vi "http transmit response.vi"(8 "error in":errorcluster, 10 "application request":T1, 11 "tcp connection":refnum<k5>) -> (0 "error out":errorcluster)   [LabVIEW 2013]
uses:
  http response.ctl
  http response packet type.ctl
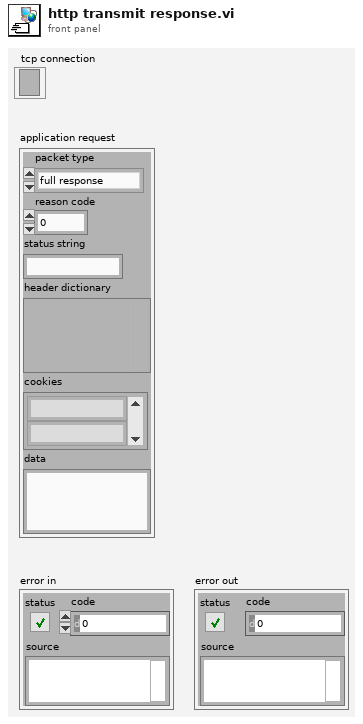
[diagram p1: front panel]
types:
  T1 = typedef "http response.ctl" = cluster{"packet type":T2, "reason code":u16, "status string":string, "header dictionary":variant, "cookies":string[], "data":string}
  T2 = typedef "http response packet type.ctl" = enum16{"full response", "header only", "data only", "last data"}
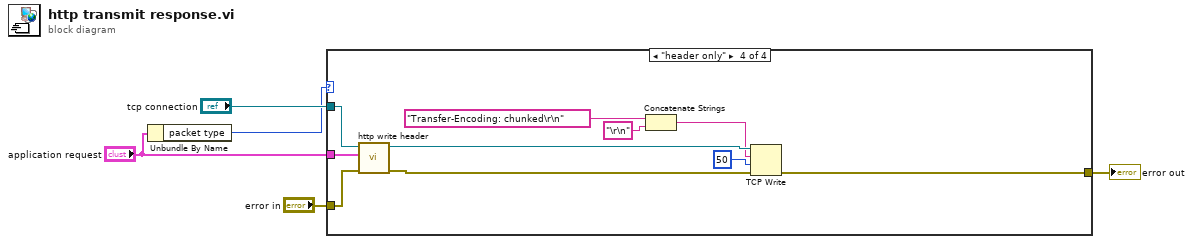
[diagram p0: block diagram]
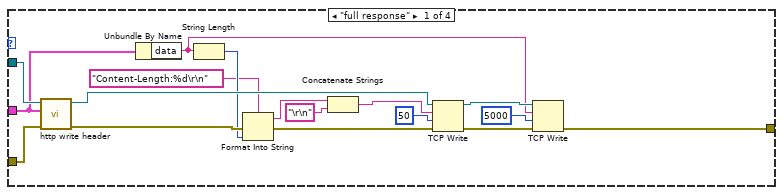
[diagram p2: hidden frame]
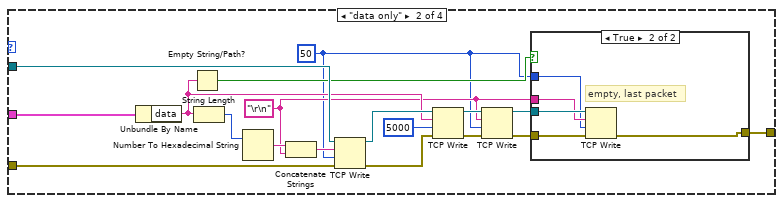
[diagram p3: hidden frame]
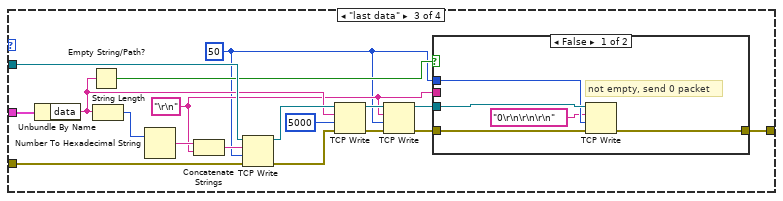
[diagram p5: hidden frame]
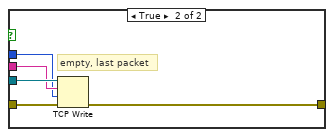
[diagram p6: hidden frame]
diagram:
  n1 = Unbundle By Name("application request") -> ("packet type"=w1:T2)
  n2 = case shown="\"header only\"" w1 {
    tunnel: "tcp connection" -> [w22 w35 w59 w84]
    tunnel: [w12 w25 w49 w79] -> w4
    tunnel: "error in" -> [w9 w40 w64 w81]
    tunnel: "application request" -> [w8 w37 w61 w80]
    frame "full response" {
      n3 = call "http write header.vi"("error in (no error)"=w9, "application request"=w8, "TCP Network Connection in"=w22) -> ("error out"=w20:errorcluster, "TCP Network Connection out"=w21:refnum<k5>)  [unwired: 7 in]
      n4 = Unbundle By Name(w8) -> ("data"=w10:string)
      n5 = String Length(string=w10) -> (length=w18:i32)
      n6 = Format Into String(format string="Content-Length:%d\r\n", error in=w20, w18) -> (resulting string=w16:string, error out=w19:errorcluster)  [unwired: 1 in]
      n7 = Concatenate Strings(w16, "\r\n" ("format string")) -> (w7:string)
      n8 = TCP Write(connection ID=w21, data in=w7, error in (no error)=w19, 9:50 ("timeout ms (25000)")) -> (connection ID out=w15:refnum<k5>, error out=w14:errorcluster)  [unwired: 1 out]
      n9 = TCP Write(connection ID=w15, data in=w10, error in (no error)=w14, 9:5000 ("timeout ms (25000)")) -> (error out=w12:errorcluster)  [unwired: 2 out]
    }
    frame "data only" {
      w23 = 50 ("timeout ms (25000)")
      w24 = "\r\n" ("format string")
      n10 = Unbundle By Name(w37) -> ("data"=w28:string)
      n11 = Empty String/Path?(string/path=w28) -> (empty?=w29:bool)
      n12 = String Length(string=w28) -> (length=w31:i32)
      n13 = Number To Hexadecimal String(2:w31) -> (0:w32:string)  [unwired: 1 in]
      n14 = Concatenate Strings(w32, w24) -> (w33:string)
      n15 = TCP Write(connection ID=w35, data in=w33, error in (no error)=w40, 9:w23) -> (connection ID out=w34:refnum<k5>, error out=w36:errorcluster)  [unwired: 1 out]
      n16 = TCP Write(connection ID=w34, data in=w28, error in (no error)=w36, 9:5000 ("timeout ms (25000)")) -> (connection ID out=w30:refnum<k5>, error out=w38:errorcluster)  [unwired: 1 out]
      n17 = TCP Write(connection ID=w30, data in=w24, error in (no error)=w38, 9:w23) -> (connection ID out=w26:refnum<k5>, error out=w27:errorcluster)  [unwired: 1 out]
      n18 = case shown="True" w29 {
        tunnel: w27 -> [w41 w45]
        tunnel: w26 -> [_ w46]
        tunnel: [w41 w44] -> w25
        tunnel: w24 -> [_ w43]
        tunnel: w23 -> [_ w42]
        frame False {
          # "not empty, not last packet"
        }
        frame True {
          # "empty, last packet"
          n19 = TCP Write(connection ID=w46, data in=w43, error in (no error)=w45, 9:w42) -> (error out=w44:errorcluster)  [unwired: 2 out]
        }
      }
    }
    frame "last data" {
      w47 = 50 ("timeout ms (25000)")
      w48 = "\r\n" ("format string")
      n20 = Unbundle By Name(w61) -> ("data"=w52:string)
      n21 = Empty String/Path?(string/path=w52) -> (empty?=w53:bool)
      n22 = String Length(string=w52) -> (length=w55:i32)
      n23 = Number To Hexadecimal String(2:w55) -> (0:w56:string)  [unwired: 1 in]
      n24 = Concatenate Strings(w56, w48) -> (w57:string)
      n25 = TCP Write(connection ID=w59, data in=w57, error in (no error)=w64, 9:w47) -> (connection ID out=w58:refnum<k5>, error out=w60:errorcluster)  [unwired: 1 out]
      n26 = TCP Write(connection ID=w58, data in=w52, error in (no error)=w60, 9:5000 ("timeout ms (25000)")) -> (connection ID out=w54:refnum<k5>, error out=w62:errorcluster)  [unwired: 1 out]
      n27 = TCP Write(connection ID=w54, data in=w48, error in (no error)=w62, 9:w47) -> (connection ID out=w50:refnum<k5>, error out=w51:errorcluster)  [unwired: 1 out]
      n28 = case shown="False" w53 {
        tunnel: w51 -> [w69 w73]
        tunnel: w50 -> [w67 w74]
        tunnel: [w68 w72] -> w49
        tunnel: w48 -> [_ w71]
        tunnel: w47 -> [w66 w70]
        frame False {
          # "not empty, send 0 packet"
          n29 = TCP Write(connection ID=w67, data in="0\r\n\r\n\r\n", error in (no error)=w69, 9:w66) -> (error out=w68:errorcluster)  [unwired: 2 out]
        }
        frame True {
          # "empty, last packet"
          n30 = TCP Write(connection ID=w74, data in=w71, error in (no error)=w73, 9:w70) -> (error out=w72:errorcluster)  [unwired: 2 out]
        }
      }
    }
    frame "header only" {
      n31 = call "http write header.vi"("error in (no error)"=w81, "application request"=w80, "TCP Network Connection in"=w84) -> ("error out"=w78:errorcluster, "TCP Network Connection out"=w83:refnum<k5>)  [unwired: 7 in]
      n32 = Concatenate Strings("Transfer-Encoding: chunked\r\n" ("format string"), "\r\n" ("format string")) -> (w76:string)
      n33 = TCP Write(connection ID=w83, data in=w76, error in (no error)=w78, 9:50 ("timeout ms (25000)")) -> (error out=w79:errorcluster)  [unwired: 2 out]
    }
  }
  "error out" <- w4
